vi "Init from Desc.vi"(8 "error in (no error)":errorcluster, 10 "Description":string, 11 "Sensor  in":refnum<class "Sensor.lvclass">) -> (0 "error out":errorcluster, 3 "Sensor out":refnum<class "Sensor.lvclass">)   [LabVIEW 2023, in "d15.lvlib" / "Sensor.lvclass"]
uses:
  Sensor.lvclass
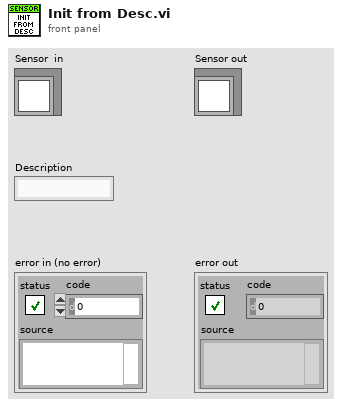
[diagram p1: front panel]
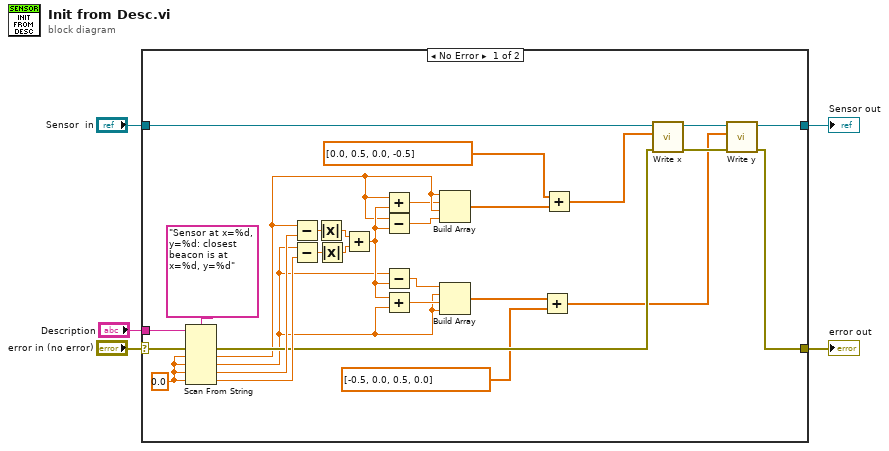
[diagram p0: block diagram]
diagram:
  n1 = case shown="No Error" "error in (no error)" {
    selector: "error in (no error)" -> [w15 w36]
    tunnel: [w30 w36] -> w4
    tunnel: [w32 w35] -> w2
    tunnel: "Sensor  in" -> [w34 w35]
    tunnel: "Description" -> [w20 _]
    frame No Error {
      w21 = 0.0 ("default value 1")
      n2 = Scan From String(format string="Sensor at x=%d, y=%d: closest beacon is at x=%d, y=%d", input string=w20, error in=w15, default 1=w21, default 2=w21, default 3=w21, default 4=w21) -> (error out=w14:errorcluster, output 1=w12:dbl, output 2=w13:dbl, output 3=w24:dbl, output 4=w23:dbl)  [unwired: 1 in, 2 out]
      n3 = Subtract(x=w12, y=w24) -> (x-y=w29:dbl)
      n4 = Subtract(x=w13, y=w23) -> (x-y=w28:dbl)
      n5 = Absolute Value(x=w29) -> (abs(x)=w27:dbl)
      n6 = Absolute Value(x=w28) -> (abs(x)=w26:dbl)
      n7 = Add(x=w27, y=w26) -> (x+y=w25:dbl)
      n8 = Add(x=w12, y=w25) -> (x+y=w11:dbl)
      n9 = Subtract(x=w12, y=w25) -> (x-y=w10:dbl)
      n10 = Subtract(x=w13, y=w25) -> (x-y=w17:dbl)
      n11 = Add(x=w25, y=w13) -> (x+y=w18:dbl)
      n12 = Build Array(w12, w11, w12, w10) -> (w19:dbl[])
      n13 = Build Array(w17, w13, w18, w13) -> (w16:dbl[])
      n14 = Add(x=w16, y=dbl[] [-0.5, 0.0, 0.5, 0.0]) -> (x+y=w7:dbl[])
      n15 = Add(x=dbl[] [0.0, 0.5, 0.0, -0.5], y=w19) -> (x+y=w9:dbl[])
      n16 = call-dynamic "Write x.vi"("error in (no error)"=w14, "x"=w9, "Diamond in"=w34) -> ("error out"=w31:errorcluster, "Diamond out"=w33:refnum<class "Sensor.lvclass">)  [unwired: 7 in]
      n17 = call-dynamic "Write y.vi"("error in (no error)"=w31, "y"=w7, "Diamond in"=w33) -> ("error out"=w30:errorcluster, "Diamond out"=w32:refnum<class "Sensor.lvclass">)  [unwired: 7 in]
    }
    frame Error {
    }
  }
  "error out" <- w4
  "Sensor out" <- w2
